vi "Mean and SD.vi"(11 "Statistics in":refnum<class "JSON Value.lvclass">) -> (1 "SD":refnum<class "JSON Scalar.lvclass">, 2 "Is SD":bool, 3 "Mean and Standard Deviation(SD)":refnum<class "JSON Value.lvclass">)   [LabVIEW 2020, in "Library Commun.lvlib" / "JSON Value.lvclass"]
uses:
  JSON Value.lvclass
  JSON Scalar/JSON Scalar.lvclass
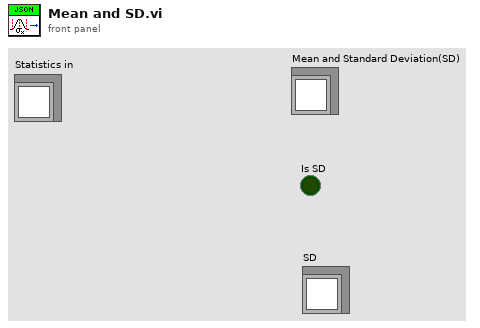
[diagram p1: front panel]
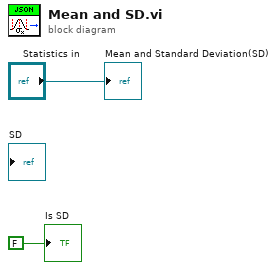
[diagram p0: block diagram]
diagram:
  "Mean and Standard Deviation(SD)" <- "Statistics in"
  "Is SD" <- FALSE ("Is SD")
